vi "bead_dropper.vi"() -> ()   [LabVIEW 2014]
panel:
  in  "Amplitude Step (mV)":dbl=1.0
  out "Current Amplitude (mV)":dbl=10.0
  out "Pulse Number":i32=1
  in  "stop":bool
  in  "Start amplitude (mV)":dbl=10.0
  in  "Stop Freq (kHz)":dbl=300.0
  in  "Start Freq (kHz)":dbl=175.0
  in  "Length of pulse (s)":dbl=1.0
  in  "Time betweeen (s)":dbl=2.0
  in  "Number of pulses":u16=40
  # "VI to pulse HP3325a generator (for use with piezo launcher)"
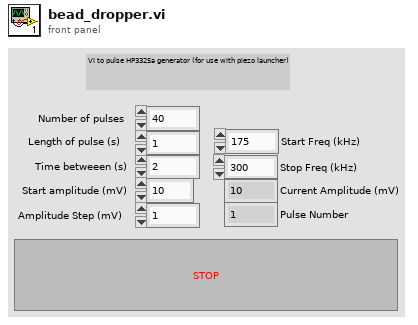
[diagram p1: front panel]
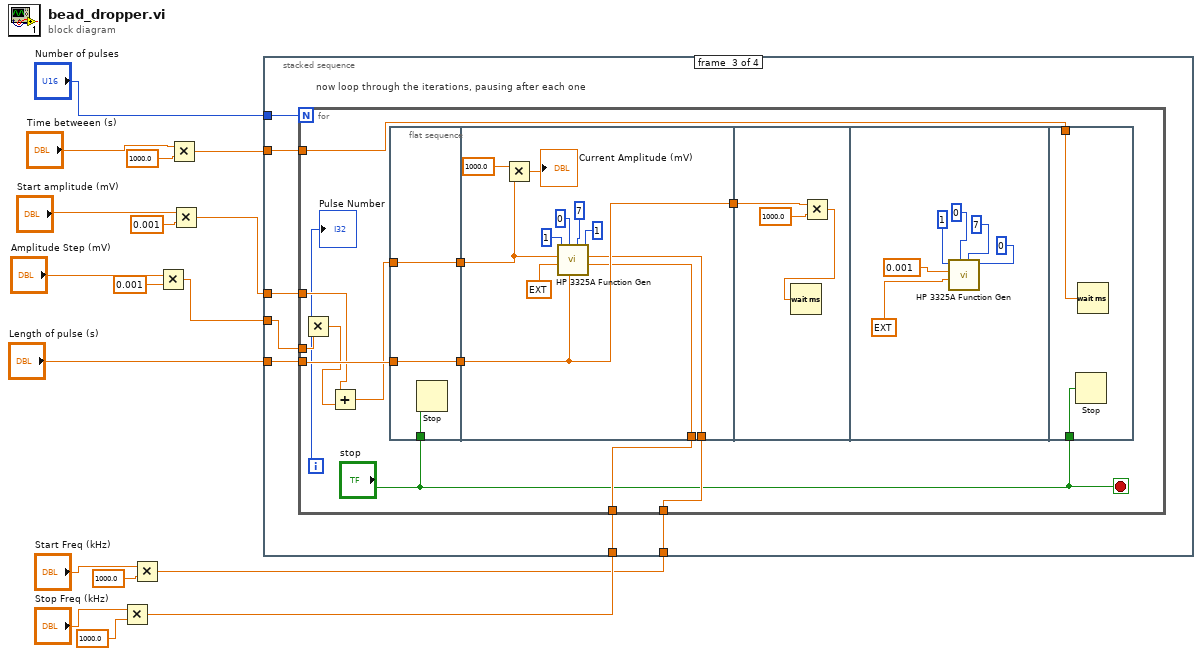
[diagram p0: block diagram]
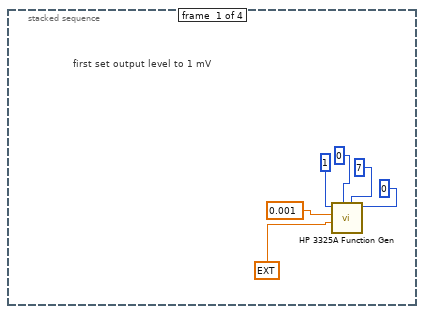
[diagram p2: hidden frame]
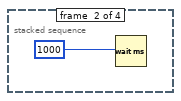
[diagram p3: hidden frame]
diagram:
  n1 = Multiply(x="Stop Freq (kHz)", y=1000.0) -> (x*y=w11:dbl)
  n2 = Multiply(x="Start Freq (kHz)", y=1000.0) -> (x*y=w10:dbl)
  n3 = Multiply(x="Amplitude Step (mV)", y=0.001) -> (x*y=w1:dbl)
  n4 = Multiply(x="Time betweeen (s)", y=1000.0) -> (x*y=w4:dbl)
  n5 = Multiply(x="Start amplitude (mV)", y=0.001) -> (x*y=w7:dbl)
  n6 = stacked-sequence {
    tunnel: "Number of pulses" -> [_ _ w31 _]
    tunnel: w7 -> [_ _ w30 _]
    tunnel: "Length of pulse (s)" -> [_ _ w29 _]
    tunnel: w11 -> [_ _ w28 _]
    tunnel: w10 -> [_ _ w27 _]
    tunnel: w4 -> [_ _ w26 _]
    tunnel: w1 -> [_ _ w25 _]
    frame #0 {
      # "first set output level to 1 mV"
      n7 = call "HP 3325A Function Gen.vi"("sweep function (none:0)"=0, "GPIB address"=7, "modulation (off:0)"=0, "offset (V)"=ext 0.0, "amplitude (V)"=0.001, "signal type (dc:0)"=i16 1) -> ()  [unwired: 6 in]
    }
    frame #1 {
      n8 = Wait (ms)(milliseconds to wait=1000) -> ()  [unwired: 1 out]
    }
    frame #2 {
      # "now loop through the iterations, pausing after each one"
      n9 = for {
        N: w31 -> [_]
        tunnel: w30 -> [w37]
        tunnel: w29 -> [w39]
        tunnel: w28 -> [w44]
        tunnel: w27 -> [w43]
        tunnel: w26 -> [w42]
        tunnel: w25 -> [w40]
        i -> [w35]
        stop <- "stop" stop-if-true
        n10 = Multiply(x=w35, y=w40) -> (x*y=w38:dbl)
        n11 = Add(x=w37, y=w38) -> (x+y=w36:dbl)
        n12 = flat-sequence {
          tunnel: w36 -> [w46]
          tunnel: w39 -> [w47]
          tunnel: [w47] -> w34
          tunnel: [w46] -> w33
          tunnel: "stop" -> [w45]
          tunnel: w44 -> [w48]
          tunnel: w43 -> [w49]
          tunnel: [w50] -> w41
          tunnel: w34 -> [w50]
          tunnel: w33 -> [w52]
          tunnel: w41 -> [w60]
          tunnel: w42 -> [w69]
          tunnel: "stop" -> [w68]
          frame #0 {
            n13 = Stop(stop? (T)=w45) -> ()
          }
          frame #1 {
            n14 = Multiply(x=1000.0, y=w52) -> (x*y=→"Current Amplitude (mV)":dbl)
            n15 = call "HP 3325A Function Gen.vi"("stop"=w48, "start"=w49, "sweep function (none:0)"=1, "GPIB address"=7, "sweep time (S)"=w50, "modulation (off:0)"=0, "offset (V)"=ext 0.0, "amplitude (V)"=w52, "signal type (dc:0)"=i16 1) -> ()  [unwired: 3 in]
          }
          frame #2 {
            n16 = Multiply(x=w60, y=1000.0) -> (x*y=w59:dbl)
            n17 = Wait (ms)(milliseconds to wait=w59) -> ()  [unwired: 1 out]
          }
          frame #3 {
            n18 = call "HP 3325A Function Gen.vi"("sweep function (none:0)"=0, "GPIB address"=7, "modulation (off:0)"=0, "offset (V)"=ext 0.0, "amplitude (V)"=0.001, "signal type (dc:0)"=i16 1) -> ()  [unwired: 6 in]
          }
          frame #4 {
            n19 = Stop(stop? (T)=w68) -> ()
            n20 = Wait (ms)(milliseconds to wait=w69) -> ()  [unwired: 1 out]
          }
        }
        "Pulse Number" <- w35
      }
    }
    frame #3 {
    }
  }
